vi "sub_check_mask_condition.vi"(10 "Current (nA)":dbl format="%#_13g", 11 "Input parameters":T1={"Measurement type"=enum."Debug", "Sensor type"=enum."HPK_8in_271ch", "Identifier"="test.txt", "Open after execution?"=FALSE, "Plot after execution?"=FALSE, "Display channel"=0, "Voltage Delay (s)"=0.5, "Switch Delay (s)"=0.01, "VISA resource name source"="", "VISA resource name DMM"="", "VISA resource name LCR"="", "Compliance  Level (A)"=10.0, "Voltage Limit (V)"=1000.0, "Data storage location"="", "Scan voltages"="", "Use source as DMM?"=FALSE, "LCR signal frequenzy (Hz)"=10.0, "DMM device"=enum."Keithley2001", "Sampling number"=1, "Use env. sensors on"=enum."Sensirion sht1x/7x", "Switchboard Handle"=0, "Use Switchboard"=FALSE, "LCR signal voltage (V)"=10000.0, "Repeat"=1, "Scan voltages IV"="", "Scan voltages CV"="", "Hex pad numbers?"=FALSE, "Set measurement type"=enum."Debug", "Custom pad scan"="", "IV voltage Delay (s)"=0.5, "CV voltage Delay (s)"=0.5, "Needle measurement?"=FALSE, "Comments"="test.txt", "LCR signal frequenzy (kHz)"=10.0, "Compliance  Level (uA)"=10.0, "Open Correction Array"=array2304x3[6912 elements], "Current set voltage"=0.0, "Last set voltage"=0.0, "Current channel"=0, "Last OpenCorrection index"=-1, "Total curr/vltg every x steps"=10, "Current channel iteration"=0, "No CV corrections"=FALSE, "Mapfile"="", "Corrfile"="", "IV voltage file"=path "", "CV voltage file"=path "", "IV Switch Delay (s)"=0.01, "CV Switch Delay (s)"=0.01, "Invert polarity"=FALSE, "Set debug dirs"=FALSE, "Is n on p"=FALSE, "Source interlock?"=TRUE, "Voltage file used?"=FALSE, "Pad mask"="", "Mask pad above (uA)"=1.0, "LCR device"=enum."LCR_E4980", "Source device"=enum."Source_2410", "HexPlot binary path"="", "PadReductionFactor"=1.0, "Temperature degC"="", "Fluence [neq]"="", "Annealing [min]"=""} {"CV Switch Delay (s)" format="%#_13g"; "IV Switch Delay (s)" format="%#_13g"; "Last set voltage" format="%#_13g"; "Current set voltage" format="%#_13g"; "CV voltage Delay (s)" format="%#_13g"; "IV voltage Delay (s)" format="%#_13g"; "Voltage Limit (V)" format="%#_13g"; "Voltage Delay (s)" format="%#_13g"; "Switch Delay (s)" format="%#_13g"}) -> (3 "Input parameters out":T1={"Measurement type"=enum."Debug", "Sensor type"=enum."HPK_8in_271ch", "Identifier"="test.txt", "Open after execution?"=FALSE, "Plot after execution?"=FALSE, "Display channel"=0, "Voltage Delay (s)"=0.5, "Switch Delay (s)"=0.01, "VISA resource name source"="", "VISA resource name DMM"="", "VISA resource name LCR"="", "Compliance  Level (A)"=10.0, "Voltage Limit (V)"=1000.0, "Data storage location"="", "Scan voltages"="", "Use source as DMM?"=FALSE, "LCR signal frequenzy (Hz)"=10.0, "DMM device"=enum."Keithley2001", "Sampling number"=1, "Use env. sensors on"=enum."Sensirion sht1x/7x", "Switchboard Handle"=0, "Use Switchboard"=FALSE, "LCR signal voltage (V)"=10000.0, "Repeat"=1, "Scan voltages IV"="", "Scan voltages CV"="", "Hex pad numbers?"=FALSE, "Set measurement type"=enum."Debug", "Custom pad scan"="", "IV voltage Delay (s)"=0.5, "CV voltage Delay (s)"=0.5, "Needle measurement?"=FALSE, "Comments"="test.txt", "LCR signal frequenzy (kHz)"=10.0, "Compliance  Level (uA)"=10.0, "Open Correction Array"=array2304x3[6912 elements], "Current set voltage"=0.0, "Last set voltage"=0.0, "Current channel"=0, "Last OpenCorrection index"=-1, "Total curr/vltg every x steps"=10, "Current channel iteration"=0, "No CV corrections"=FALSE, "Mapfile"="", "Corrfile"="", "IV voltage file"=path "", "CV voltage file"=path "", "IV Switch Delay (s)"=0.01, "CV Switch Delay (s)"=0.01, "Invert polarity"=FALSE, "Set debug dirs"=FALSE, "Is n on p"=FALSE, "Source interlock?"=TRUE, "Voltage file used?"=FALSE, "Pad mask"="", "Mask pad above (uA)"=1.0, "LCR device"=enum."LCR_E4980", "Source device"=enum."Source_2410", "HexPlot binary path"="", "PadReductionFactor"=1.0, "Temperature degC"="", "Fluence [neq]"="", "Annealing [min]"=""} {"CV Switch Delay (s)" format="%#_13g"; "IV Switch Delay (s)" format="%#_13g"; "Last set voltage" format="%#_13g"; "Current set voltage" format="%#_13g"; "CV voltage Delay (s)" format="%#_13g"; "IV voltage Delay (s)" format="%#_13g"; "Voltage Limit (V)" format="%#_13g"; "Voltage Delay (s)" format="%#_13g"; "Switch Delay (s)" format="%#_13g"})   [LabVIEW 2020]
uses:
  input_params.ctl
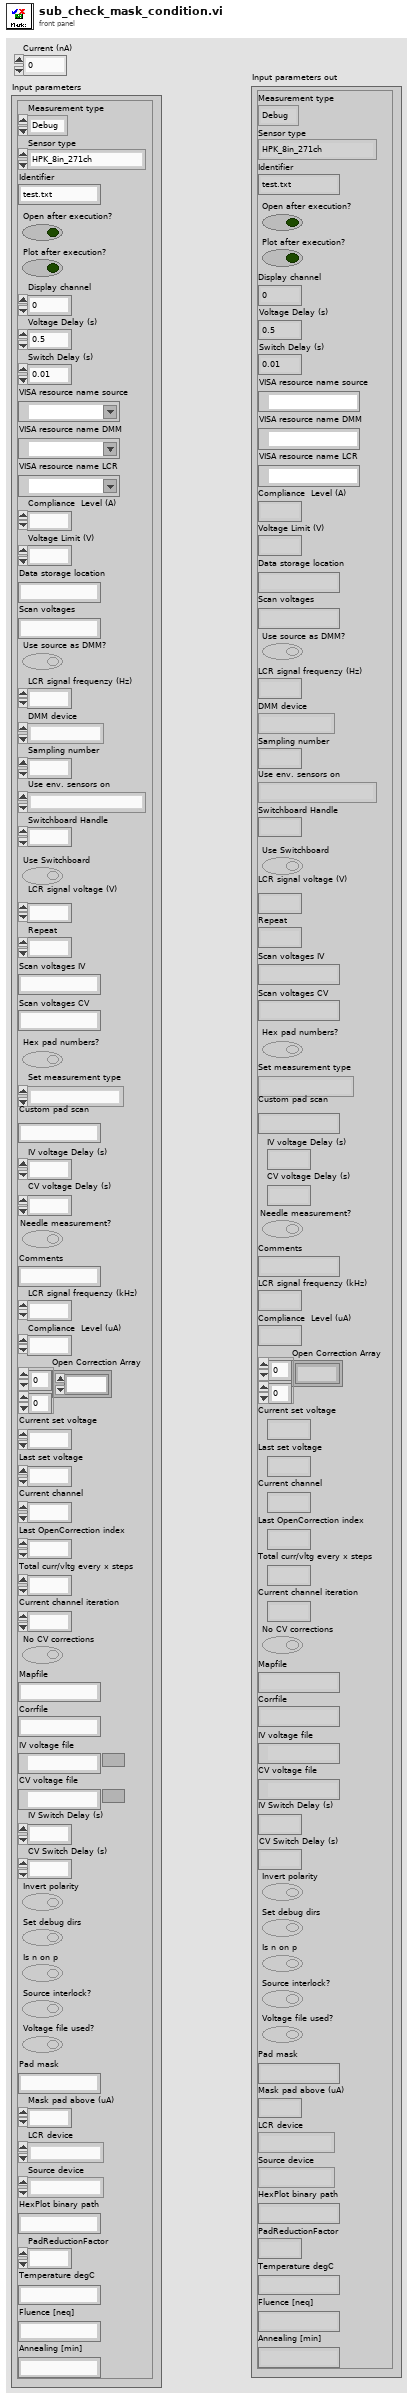
[diagram p1: front panel]
types:
  T1 = typedef "input_params.ctl" = cluster{"Measurement type":enum16{"IV", "CV", "Debug", "Test_contact"}, "Sensor type":enum16{"HPK_6in_135ch", "HPK_8in_271ch", "IFX_8in_256ch", "Diode", "HPK_6in_239ch", "Full_Matrix", "HPK_8in_271ch_full", "LumiCal", "HPK_8in_444ch", "HPK_8in_198ch_2019", "HPK_8in_MGW_LD_full", "HPK_8in_MGW_LD_a_type_top", "HPK_8in_MGW_LD_a_type_bottom", "HPK_8in_MGW_LD_b_type_left", "HPK_8in_MGW_LD_b_type_right", "HPK_8in_MGW_LD_c_type_left", "HPK_8in_MGW_LD_c_type_right", "HPK_8in_MGW_HD_full", "HPK_8in_MGW_HD_a_type_top", "HPK_8in_MGW_HD_a_type_bottom", "HPK_8in_MGW_HD_b_type_left", "HPK_8in_MGW_HD_b_type_right", "HPK_8in_MGW_HD_c_type_left", "HPK_8in_MGW_HD_c_type_right", "CALICE_6in_256ch"}, "Identifier":string, "Open after execution?":bool, "Plot after execution?":bool, "Display channel":i32, "Voltage Delay (s)":dbl, "Switch Delay (s)":dbl, "VISA resource name source":refnum<visa-resource-name>, "VISA resource name DMM":refnum<visa-resource-name>, "VISA resource name LCR":refnum<visa-resource-name>, "Compliance  Level (A)":dbl, "Voltage Limit (V)":dbl, "Data storage location":string, "Scan voltages":string, "Use source as DMM?":bool, "LCR signal frequenzy (Hz)":dbl, "DMM device":enum16{"Keithley2001", "Keithley2450", "Keithley2410", "Keithley6485", "Keithley6487", "Keithley6517"}, "Sampling number":i32, "Use env. sensors on":enum16{"Sensirion sht1x/7x", "Switch Matrix", "Probecard"}, "Switchboard Handle":u32, "Use Switchboard":bool, "LCR signal voltage (V)":dbl, "Repeat":i32, "Scan voltages IV":string, "Scan voltages CV":string, "Hex pad numbers?":bool, "Set measurement type":enum16{"IV", "CV", "Debug", "Test_contact", "IV+CV"}, "Custom pad scan":string, "IV voltage Delay (s)":dbl, "CV voltage Delay (s)":dbl, "Needle measurement?":bool, "Comments":string, "LCR signal frequenzy (kHz)":dbl, "Compliance  Level (uA)":dbl, "Open Correction Array":dbl[][], "Current set voltage":dbl, "Last set voltage":dbl, "Current channel":i32, "Last OpenCorrection index":i32, "Total curr/vltg every x steps":i32, "Current channel iteration":i32, "No CV corrections":bool, "Mapfile":string, "Corrfile":string, "IV voltage file":path, "CV voltage file":path, "IV Switch Delay (s)":dbl, "CV Switch Delay (s)":dbl, "Invert polarity":bool, "Set debug dirs":bool, "Is n on p":bool, "Source interlock?":bool, "Voltage file used?":bool, "Pad mask":string, "Mask pad above (uA)":dbl, "LCR device":enum16{"LCR_E4980", "AGILENT_4263X"}, "Source device":enum16{"Source_2410", "Source_6487"}, "HexPlot binary path":string, "PadReductionFactor":dbl, "Temperature degC":string, "Fluence [neq]":string, "Annealing [min]":string}
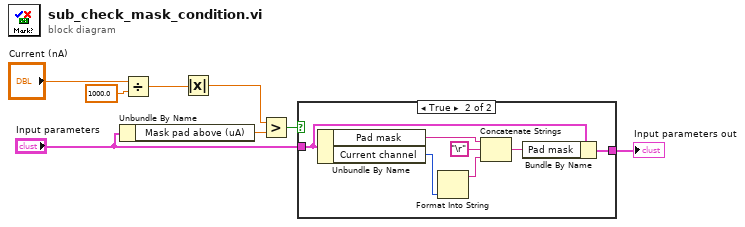
[diagram p0: block diagram]
diagram:
  n1 = Unbundle By Name("Input parameters") -> ("Mask pad above (uA)"=w8:dbl)
  n2 = Divide(x="Current (nA)", y=1000.0) -> (x/y=w2:dbl)
  n3 = Absolute Value(x=w2) -> (abs(x)=w1:dbl)
  n4 = Greater?(x=w1, y=w8) -> (0:w5:bool)
  n5 = case shown="True" w5 {
    tunnel: "Input parameters" -> [w9 w11]
    tunnel: [w9 w10] -> w3
    frame False {
    }
    frame True {
      n6 = Unbundle By Name(w11) -> ("Pad mask"=w16:string, "Current channel"=w14:i32)
      n7 = Format Into String(w14) -> (resulting string=w13:string)  [unwired: 3 in, 1 out]
      n8 = Concatenate Strings(w16, "\r", w13) -> (w12:string)
      n9 = Bundle By Name(cluster=w11, "Pad mask"=w12) -> (w10:T1)
    }
  }
  "Input parameters out" <- w3
